vi "sv_Peak View Harmonics (Continuous Swept).vi"(7 "harmonic units":T7(ring), 8 "error in (no error)":errorcluster, 9 "spectrum info":T1={"channel name"="", "description"="", "x-axis units"=0, "spectral info"={"spectrum type"=enum."Power [Magnitude^2]", "linear/dB"=enum."linear", "window"=0, "window size"=0, "FFT size"=0}, "engineering units"=0, "custom label"="", "dB reference [EU]"=0.0, "peak units"=enum."rms", "weighting filter"=0, "spectral density?"=FALSE, "unit label"="", "spectrum skewed?"=FALSE, "complimentary spectrum units"=enum."none"} {"x-axis units" items=["Time (s)"=0, "Frequency-CB (Hz)"=1, "Frequency-CPB (Hz)"=1248, "Frequency-Arbitrary (Hz)"=2357, "Quefrency (s)"=2, "Revolutions (rev)"=3, "Order"=4, "Speed (RPM)"=11, "Speed (rad/s)"=21, "Index"=65535]; "weighting filter" items=["Linear", "A-weighting", "B-weighting", "C-weighting", "ITU-R 468-4", "Dolby", "CCITT", "C-message", "Wb", "Wc", "Wd", "We", "Wf", "Wh", "Wj", "Wk", "Wm", "AES17 20 kHz lowpass", "AES17 40 kHz lowpass", "AES17 20 kHz highpass", "AES17 40 kHz highpass"]; "dB reference [EU]" format="%.2f"; "engineering units" items=["custom..."=0, "V"=1, "A"=21, "C"=30, "pC"=31, "s"=32, "-"=29, "Pa"=2, "N"=20, "g"=3, "m/s^2"=4, "m/s"=5, "m"=6, "mm/s"=12, "mm"=13, "micron/s"=14, "micron"=15, "in/s^2"=7, "in/s"=8, "in"=9, "mil/s"=10, "mil"=11, "rad/s^2"=16, "rad/s"=17, "rad"=18, "deg/s^2"=26, "deg/s"=27, "deg"=28, "RPM"=22, "cycle/s^2"=23, "Hz"=24, "cycle"=25, "strain"=19]; "spectral info"."window" items=["None "=0, "Hanning"=1, "Hamming"=2, "Blackman-Harris"=3, "Exact Blackman"=4, "Blackman"=5, "Flat Top"=6, "4 Term B-Harris "=7, "7 Term B-Harris"=8, "Low Sidelobe"=9, "Force - Exponential"=10, "Gaussian"=62]}, 10 "fundamental amplitude [EU rms]":dbl[](array[numeric]) format="%.2f", 11 "harmonic amplitudes [EU rms]":dbl[](array[numeric]) format="%.2f") -> (0 "error out":errorcluster, 3 "converted harmonic amplitudes":dbl[](array[numeric]) format="%.2f", 5 "unit label":string)   [LabVIEW 2017, in "SoundVib_ContSweptSine.lvlib"]
uses:
  <vilib>/addons/Sound and Vibration/svt_Continuous Swept Sine/SoundVib_ContSweptSine.lvlib
  <vilib>/addons/_NISVFA/_Shared subVIs/Controls/svc_Spectrum Info.ctl
  <vilib>/addons/_NISVFA/_Shared subVIs/Controls/svc_X-Axis Units.ctl
  <vilib>/addons/_NISVFA/_Shared subVIs/Controls/svc_Spectrum Type.ctl
  <vilib>/addons/_NISVFA/_Shared subVIs/Controls/svc_Engineering Units Text Ring.ctl
  <vilib>/addons/_NISVFA/_Shared subVIs/Controls/svc_Weighting Filter Text Ring.ctl
  <vilib>/addons/_NISVFA/_Shared subVIs/Controls/svc_Complimentary Spectrum Units.ctl
  <vilib>/addons/_NISVFA/_Shared subVIs/Common/svc_Get Weighting Enum and Labels.vi
  <vilib>/addons/_NISVFA/_Shared subVIs/Common/svc_Unit Label Lexical Class.vi
  <vilib>/addons/_NISVFA/_Shared subVIs/Common/svc_Engineering Units to Unit Label.vi
  <vilib>/addons/_NISVFA/_Shared subVIs/Common/svc_Format Value (DBL).vi
  <vilib>/addons/Sound and Vibration/svt_Distortion/SoundVib_Distortion.lvlib
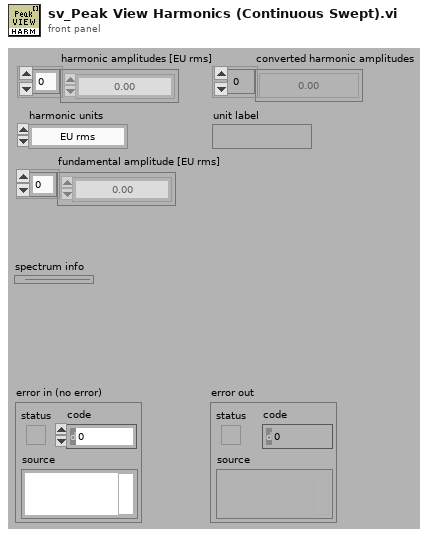
[diagram p1: front panel]
types:
  T1 = typedef "svc_Spectrum Info.ctl" = cluster{"channel name":string, "description":string, "x-axis units":T2, "spectral info":cluster{"spectrum type":T3, "linear/dB":enum16{"linear", "dB"}, "window":u16, "window size":i32, "FFT size":i32}, "engineering units":T4, "custom label":string, "dB reference [EU]":dbl, "peak units":enum16{"rms", "peak", "peak-peak"}, "weighting filter":T5, "spectral density?":bool, "unit label":string, "spectrum skewed?":bool, "complimentary spectrum units":T6}
  T2 = typedef "svc_X-Axis Units.ctl" = u16
  T3 = typedef "svc_Spectrum Type.ctl" = enum16{"FFT Spectrum [complex]", "Amplitude [Magnitude]", "Power [Magnitude^2]", "Cross Spectrum [complex]", "Frequency Response [Complex]"}
  T4 = typedef "svc_Engineering Units Text Ring.ctl" = u16
  T5 = typedef "svc_Weighting Filter Text Ring.ctl" = u16
  T6 = typedef "svc_Complimentary Spectrum Units.ctl" = enum16{"none", "radians", "degrees", "cycles", "imaginary"}
  T7 = enum16{"EU rms", "EU peak", "EU peak-peak", "dB ref fund"}
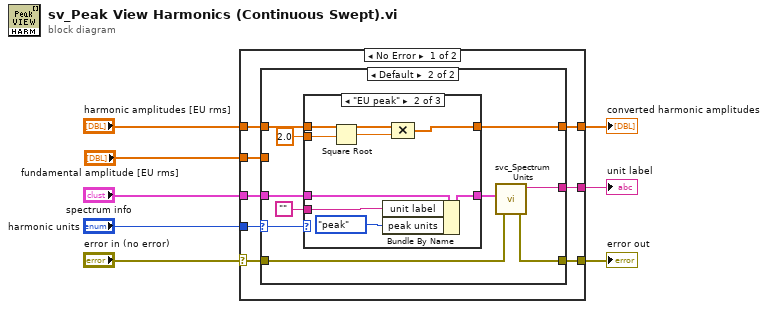
[diagram p0: block diagram]
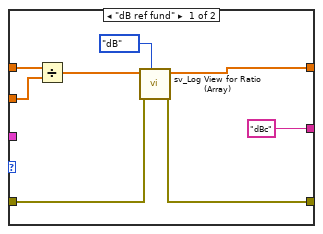
[diagram p2: hidden frame]
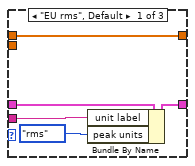
[diagram p3: hidden frame]
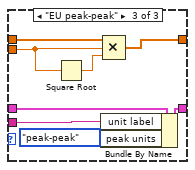
[diagram p4: hidden frame]
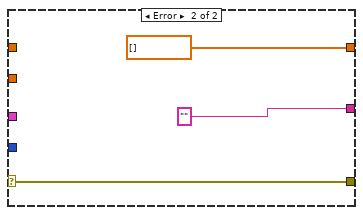
[diagram p5: hidden frame]
diagram:
  n1 = case shown="No Error" "error in (no error)" {
    selector: "error in (no error)" -> [w12 w56]
    tunnel: [w13 ""] -> w8
    tunnel: [w16 dbl[] [] ("peak amplitudes [EU pk]")] -> w2
    tunnel: "harmonic amplitudes [EU rms]" -> [w15 _]
    tunnel: "harmonic units" -> [w10 _]
    tunnel: [w11 w56] -> w5
    tunnel: "spectrum info" -> [w14 _]
    tunnel: "fundamental amplitude [EU rms]" -> [w9 _]
    frame No Error {
      n2 = case shown="Default" w10 {
        selector: w10 -> [_ w26]
        tunnel: [w18 w33] -> w16
        tunnel: w15 -> [w22 w32]
        tunnel: w14 -> [_ w31]
        tunnel: ["dBc" ("unit label") w29] -> w13
        tunnel: w12 -> [w24 w28]
        tunnel: [w23 w27] -> w11
        tunnel: w9 -> [w21 _]
        frame "dB ref fund" {
          n3 = Divide(x=w22, y=w21) -> (x/y=w20:dbl[])
          n4 = call <vilib>:"sv_Log View for Ratio (Array).vi"("ratio units"=enum16{"dB", "linear ratio", "%"}."dB", "error in (no error)"=w24, "linear ratio"=w20) -> ("error out"=w23:errorcluster, "converted ratio"=w18:dbl[])  [unwired: 6 in, 1 out]
        }
        frame Default {
          n5 = case shown="\"EU peak\"" w26 {
            tunnel: w32 -> [w35 w47 w55]
            tunnel: [w35 w42 w54] -> w33
            tunnel: 2.0 ("y") -> [_ w41 w48]
            tunnel: w31 -> [w39 w45 w52]
            tunnel: [w37 w44 w51] -> w30
            tunnel: "" -> [w36 w43 w50]
            frame "EU rms", Default {
              n6 = Bundle By Name(cluster=w39, "unit label"=w36, "peak units"=enum16{"rms", "peak", "peak-peak"}."rms") -> (w37:T1)
            }
            frame "EU peak" {
              n7 = Square Root(x=w41) -> (sqrt(x)=w40:dbl)
              n8 = Bundle By Name(cluster=w45, "unit label"=w43, "peak units"=enum16{"rms", "peak", "peak-peak"}."peak") -> (w44:T1)
              n9 = Compound Arithmetic op=MULTIPLY(w47, w40) -> (w42:dbl[])
            }
            frame "EU peak-peak" {
              n10 = Square Root(x=w48) -> (sqrt(x)=w49:dbl)
              n11 = Bundle By Name(cluster=w52, "unit label"=w50, "peak units"=enum16{"rms", "peak", "peak-peak"}."peak-peak") -> (w51:T1)
              n12 = Compound Arithmetic op=MULTIPLY(w55, w48, w49) -> (w54:dbl[])
            }
          }
          n13 = call <vilib>:"svc_Spectrum Units.vi"("error in (no error)"=w28, "spectrum info in"=w30) -> ("error out"=w27:errorcluster, "unit label"=w29:string)  [unwired: 2 in, 2 out]
        }
      }
    }
    frame Error {
    }
  }
  "unit label" <- w8
  "error out" <- w5
  "converted harmonic amplitudes" <- w2
